vi "Control Panel.vi"(8 "error in (no error)":errorcluster, 11 "Photon Counter SR400 bogus in":refnum<class "Photon Counter SR400.lvclass">) -> (0 "error out":errorcluster, 3 "Photon Counter SR400 bogus out":refnum<class "Photon Counter SR400.lvclass">)   [LabVIEW 2012, in "Photon Counter SR400.lvclass"]
uses:
  Photon Counter SR400.lvclass
  SR400/Public/Typedefs.llb/Gate Mode.ctl
  Photon Counter SR400.lvclass/Photon Counter SR400.ctl
  SR400/SR400.lvlib
  Utility Classes/Readable/Readable.lvclass
panel:
  out "Update visible/hidden":bool
  out "Gate B Mode":T1
  out "Gate A Mode":T1
  in  "stop":bool
  in  "Read to Control":bool
  in  "Read":bool
  in  "Initialize":bool
  out "Gate A % Current":dbl
  out "Gate B % Current":dbl
  in  "Gate B % Set":dbl
  in  "Gate A % Set":dbl
  in  "Gate Width: Time / Percent":bool caption="Gate Width\n        Time / Percent"
  in  "Gate Delay Reference\n        Start / Middle":bool
  in  "Gate B Mode Set":T1
  in  "Gate A Mode Set":T1
  out "Trigger Freq Current":dbl[unit]=42077.399999999994 caption="Trigger Freq"
  in  "Trigger Freq Set":dbl[unit]=42077.399999999994 caption="Trigger Freq."
  in  "Set Time & Freq.":bool
  in  "# Triggers vs Freq/Time":bool
  out "# of Cycles Current":dbl format="%^#_6g"
  in  "# of Cycles Set":dbl format="%^#_6g"
  in  "Set # of Triggers":bool
  in  "Internal / External":bool
  out "cpsB":dbl[unit] caption="CPS B"
  out "cpsA":dbl[unit] caption="CPS A"
  in  "Gate B Width Set":dbl[unit] caption="Gate B Width"
  in  "Gate A Width Set":dbl[unit]
  out "Gate A Width":dbl[unit] format="%^#_6g"
  out "Gate B Width":dbl[unit] format="%^#_6g"
  out "Gate B Delay":dbl[unit]
  out "Gate A Delay":dbl[unit]
  in  "Gate B Delay Set":dbl[unit]
  in  "Gate A Delay Set":dbl[unit]
  in  "Set Gate Delays":bool
  in  "Set Gate Mode":bool
  in  "Set Gate Widths":bool
  in  "Read Channels":bool
  in  "Count Time Set":dbl[unit]
  out "Count Time Current":dbl[unit]=1.0 min=0.0 max=10000.0 step=1.0 format="%#_7g"
  in  "Set Count Time":bool
  out "Photon Counter SR400":refnum<class "Photon Counter SR400.lvclass">
  # "Gates"
  # "Trigger"
  # "Gate A"
  # "Gate B"
  # "Channels"
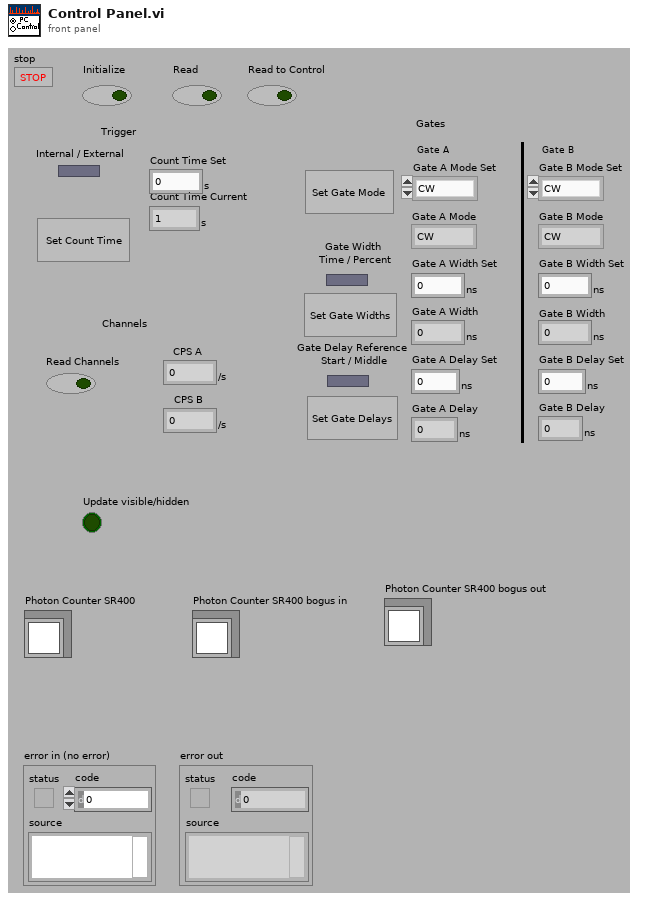
[diagram p1: front panel]
types:
  T1 = typedef "SR400.lvlib/Gate Mode.ctl" = enum16{"CW", "Fixed", "Scan"}
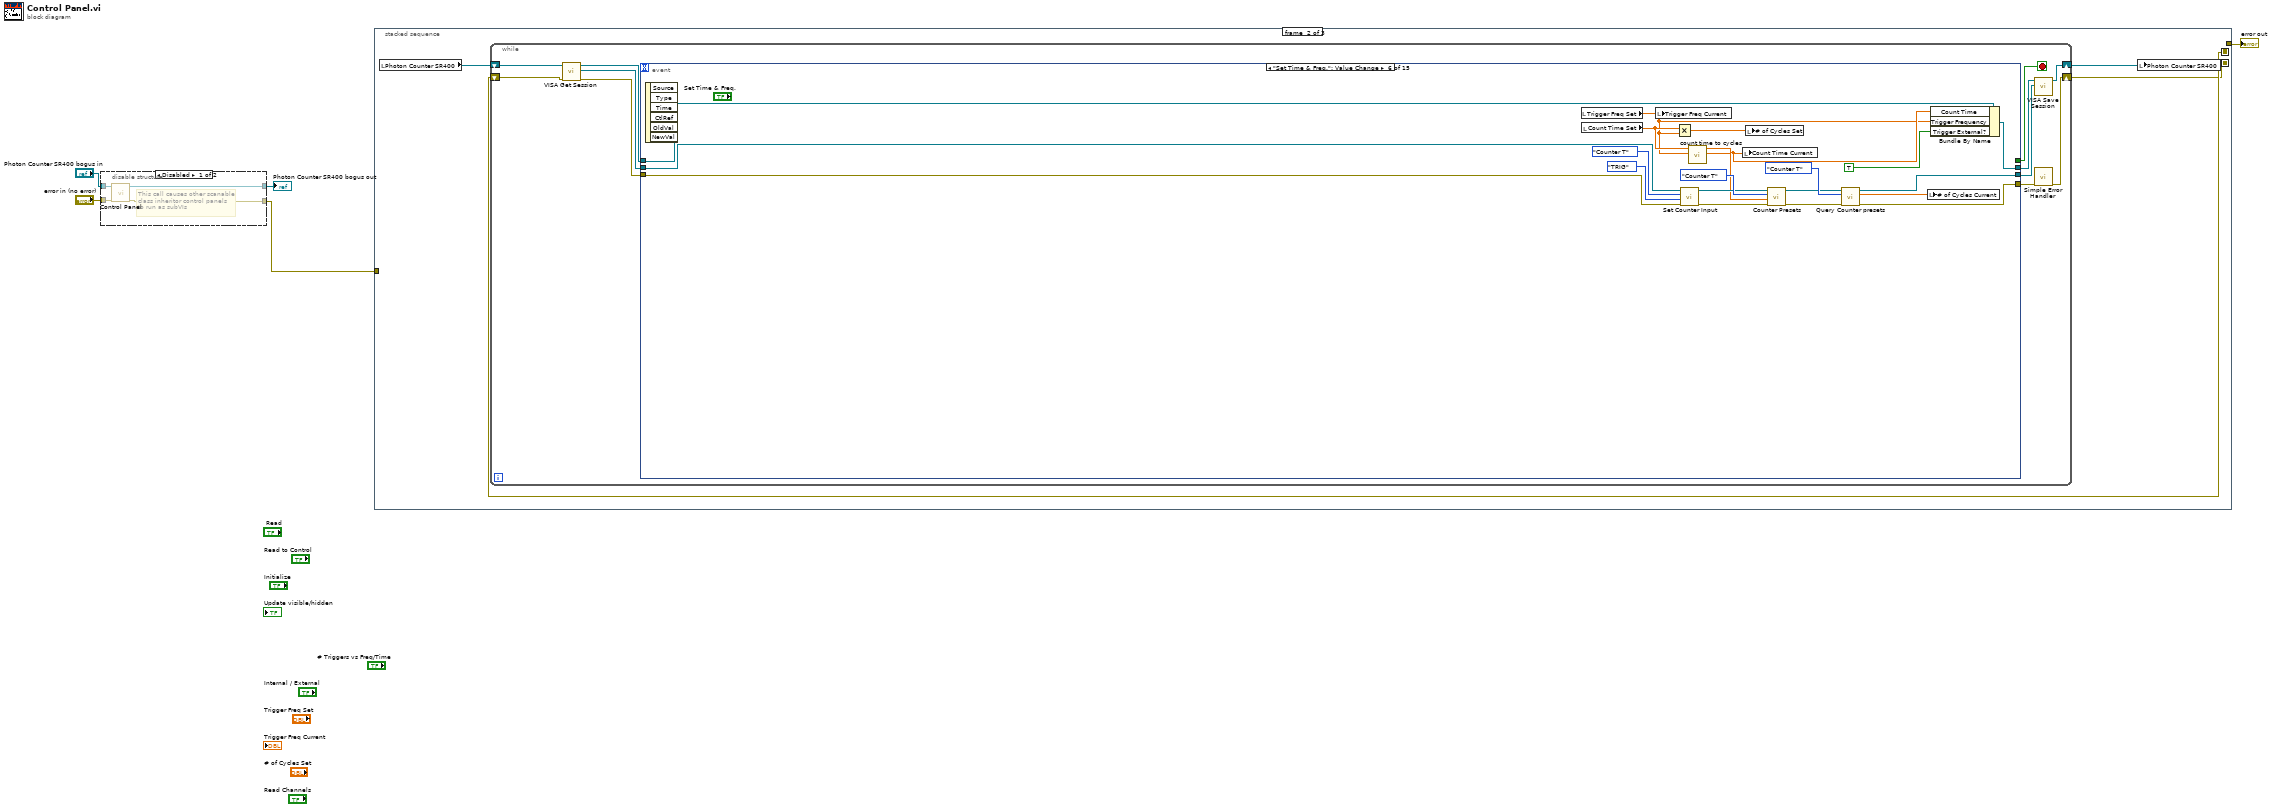
[diagram p0: block diagram]
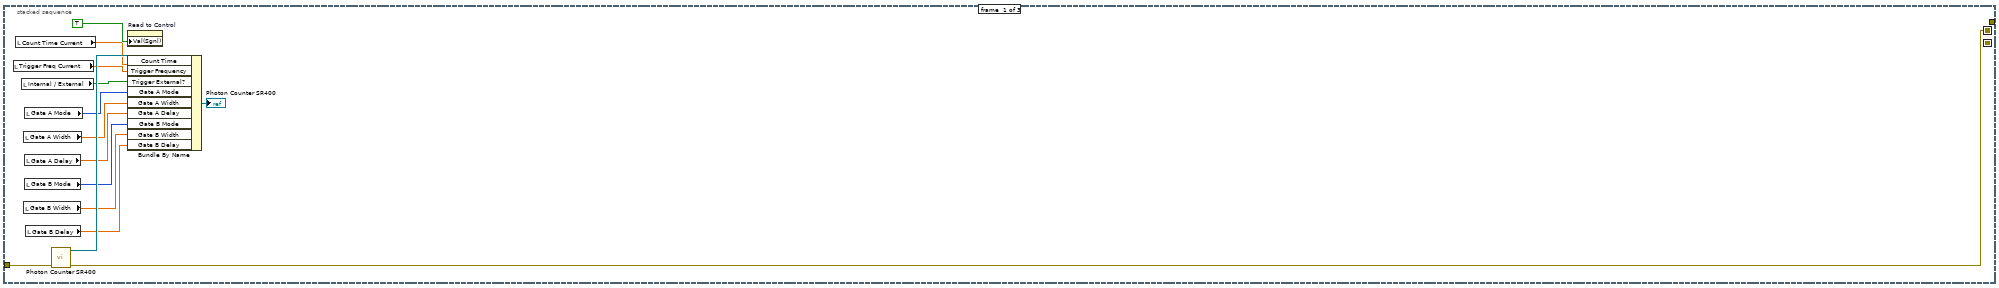
[diagram p3: hidden frame]
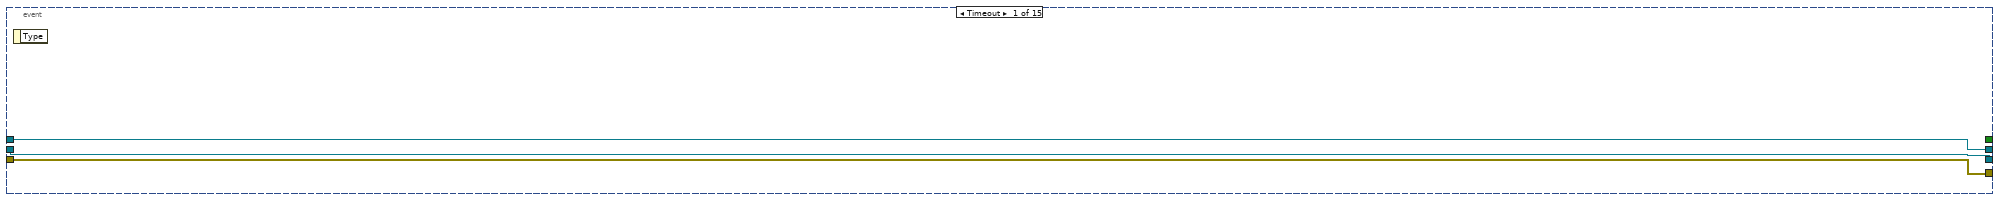
[diagram p4: hidden frame]
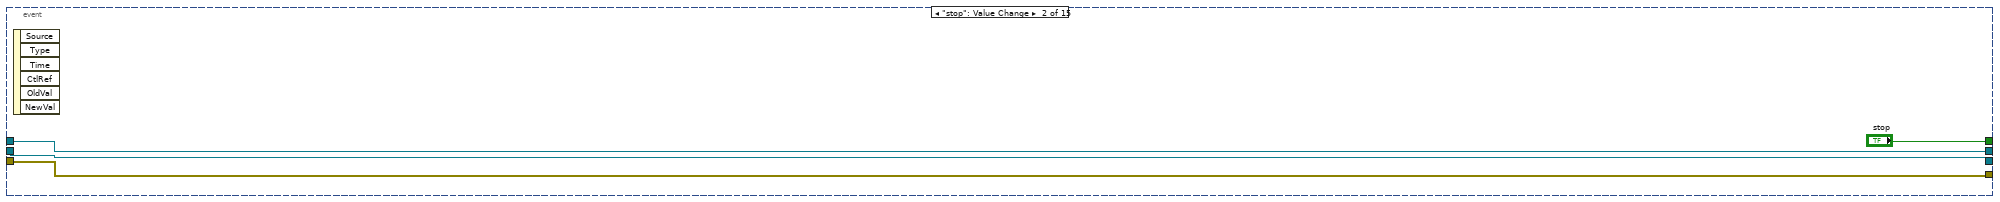
[diagram p5: hidden frame]
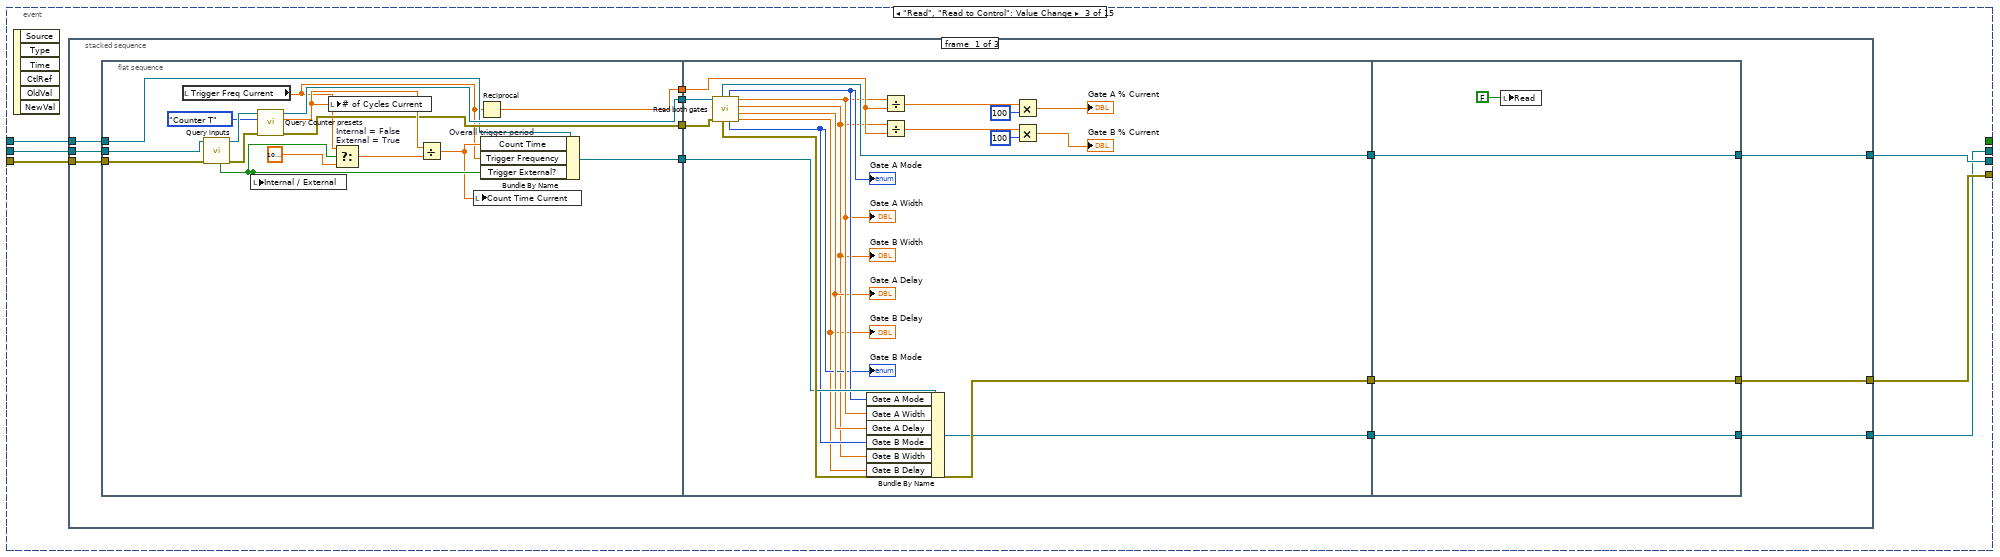
[diagram p6: hidden frame]
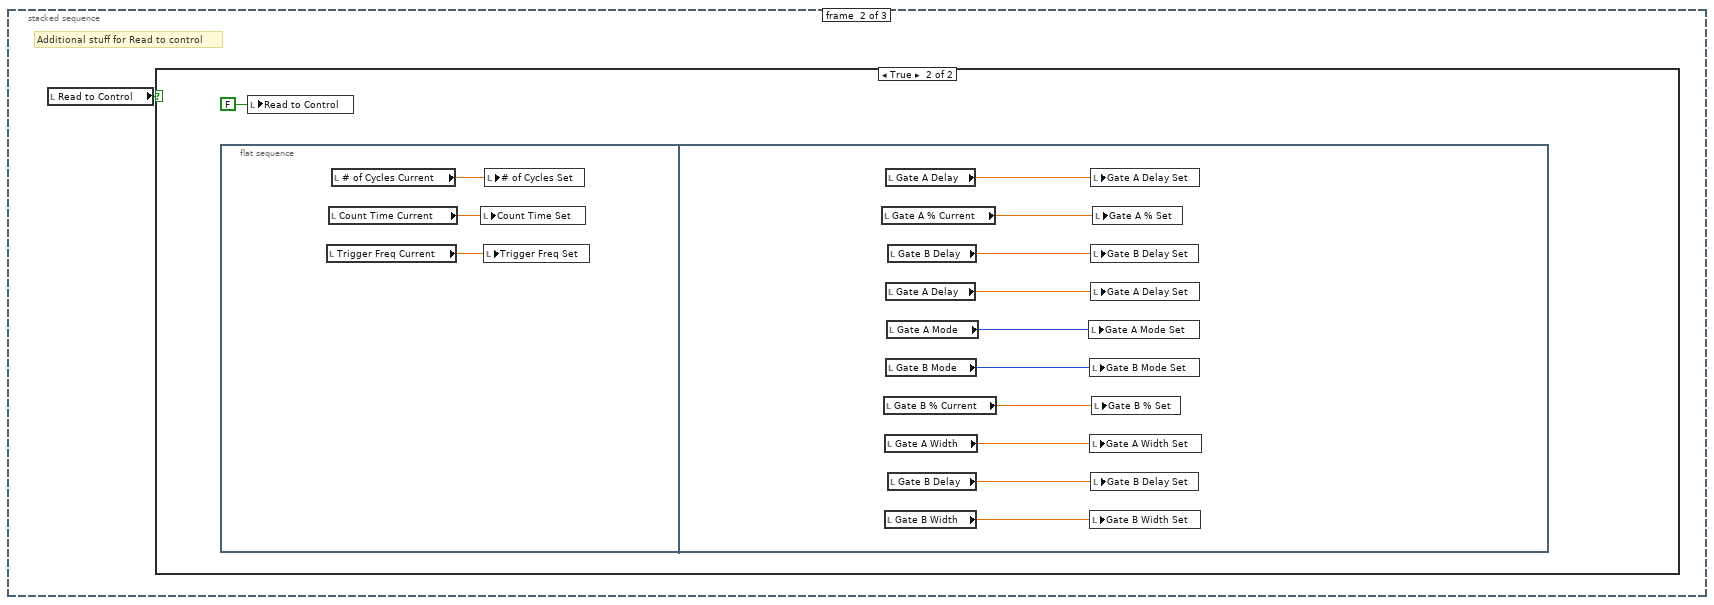
[diagram p7: hidden frame]
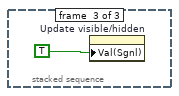
[diagram p9: hidden frame]
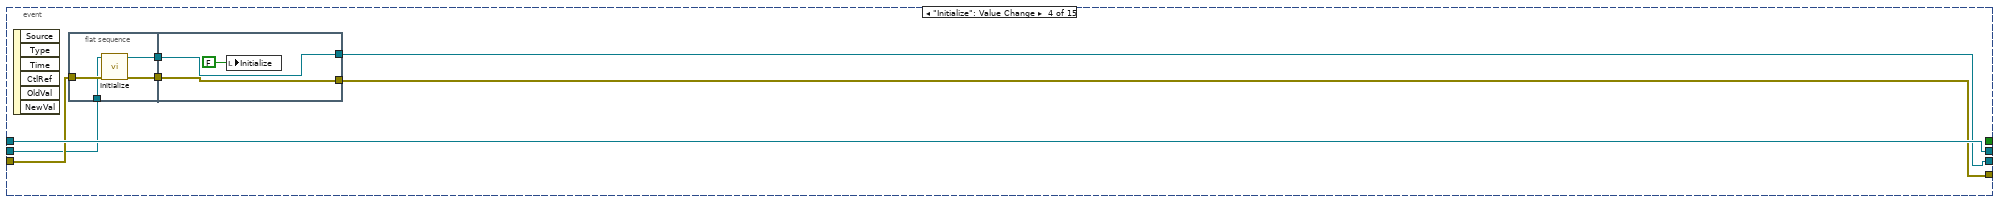
[diagram p10: hidden frame]
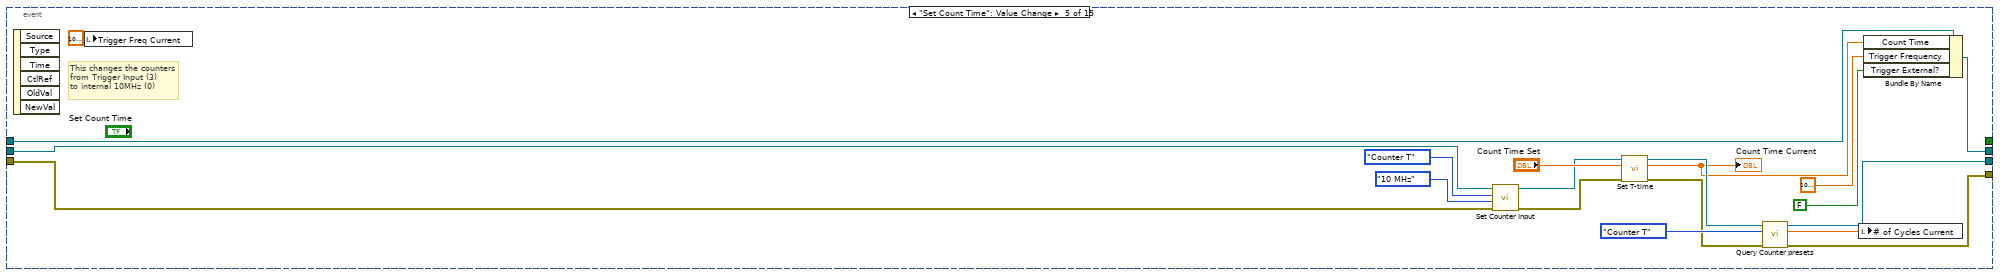
[diagram p11: hidden frame]
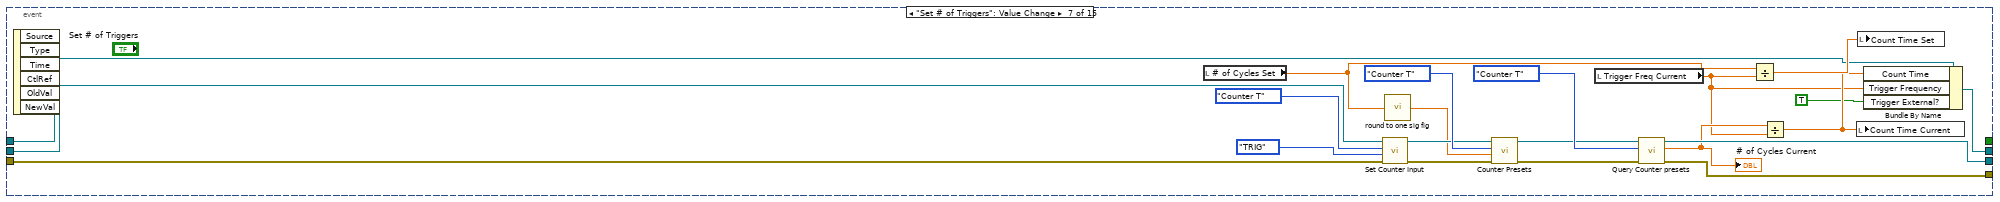
[diagram p12: hidden frame]
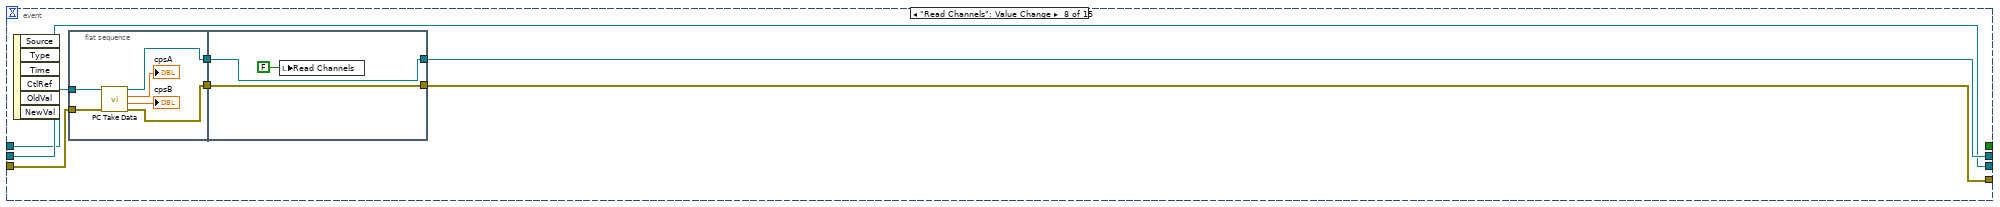
[diagram p13: hidden frame]
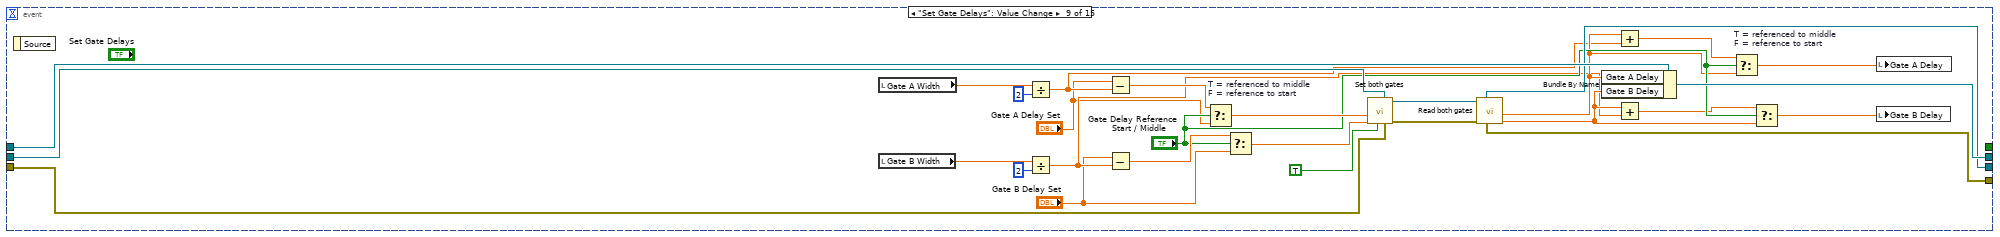
[diagram p14: hidden frame]
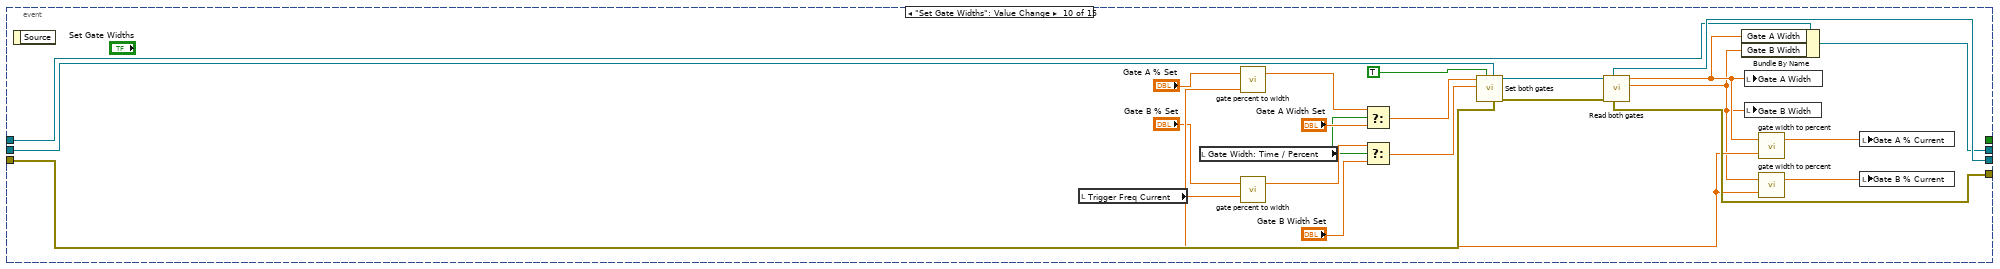
[diagram p15: hidden frame]
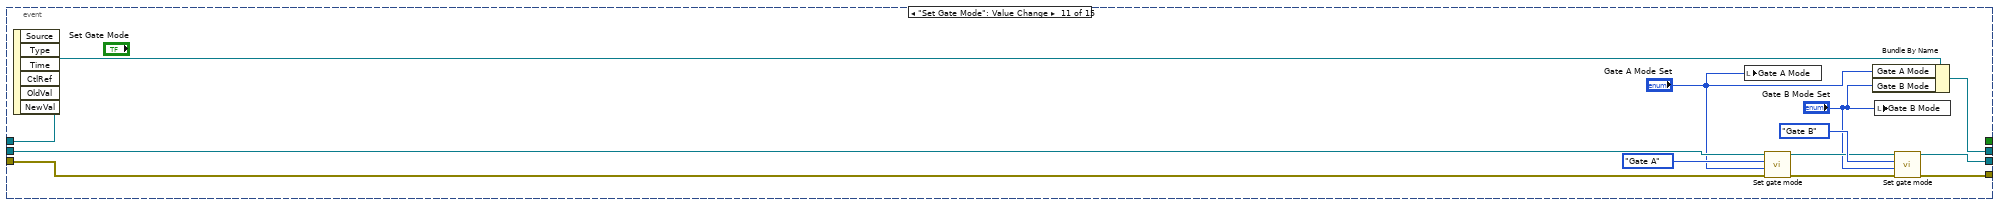
[diagram p16: hidden frame]
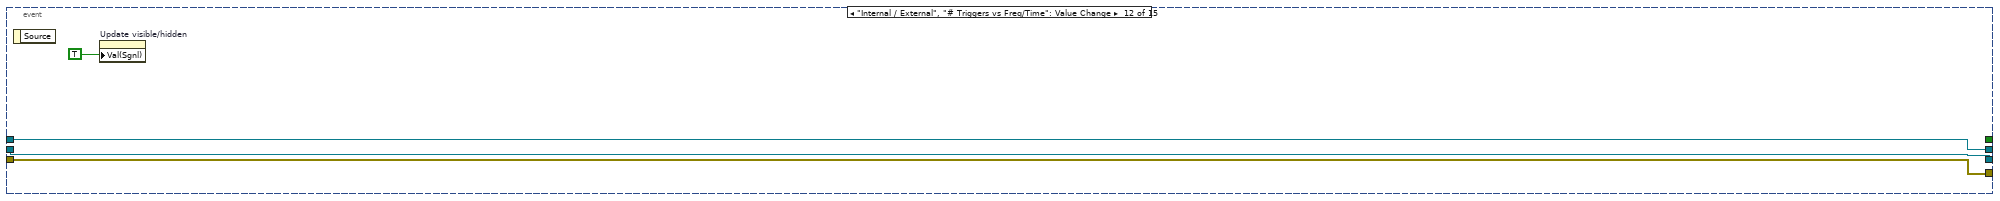
[diagram p17: hidden frame]
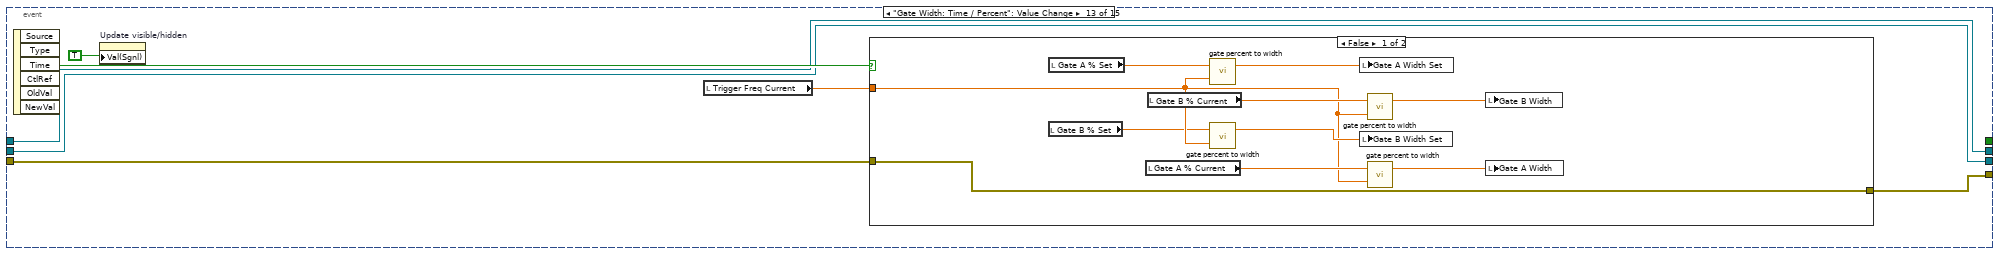
[diagram p18: hidden frame]
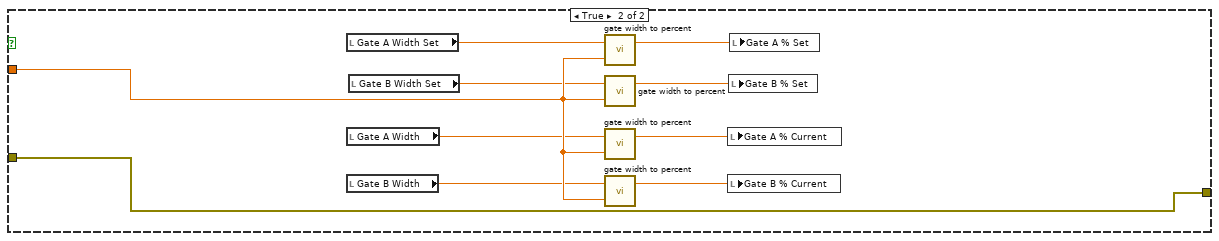
[diagram p19: hidden frame]
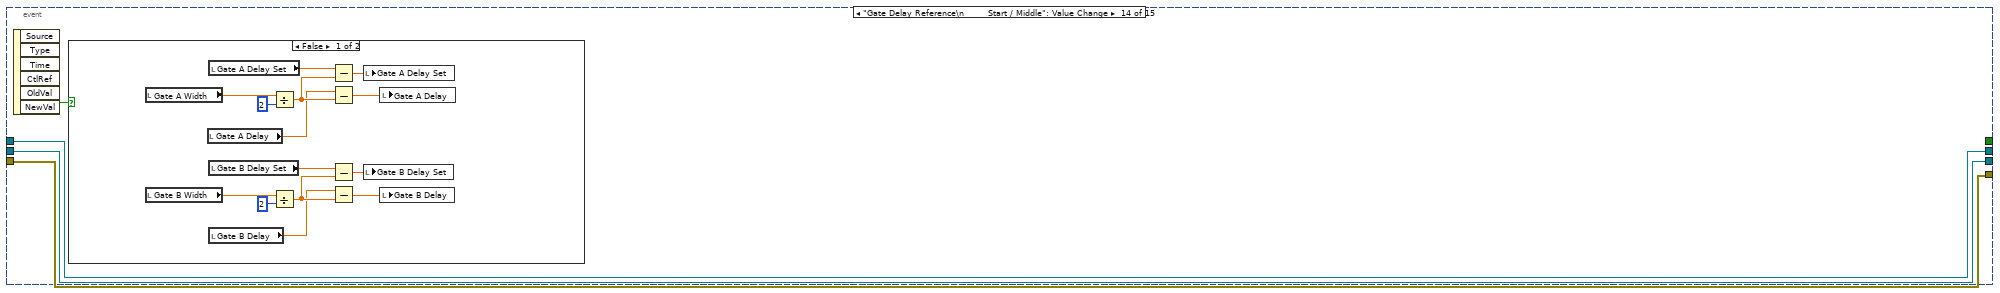
[diagram p20: hidden frame]
diagram:
  n1 = disable-structure shown="Disabled" {
    disable-tunnel: "error in (no error)" -> [w9 w10]
    disable-tunnel: [w8 w10] -> w3
    disable-tunnel: [w7 w11] -> w2
    disable-tunnel: "Photon Counter SR400 bogus in" -> [w6 w11]
    frame Disabled {
      # "This call causes other scanable\nclass inheritor control panels\nto run as subVIs"
      n2 = call-parent "Control Panel.vi"("error in (no error)"=w9, "Instrument in"=w6) -> ("error out"=w8:errorcluster, "Instrument out"=w7:refnum<class "Photon Counter SR400.lvclass">)  [unwired: 8 in]
    }
    frame Enabled {
    }
  }
  "Photon Counter SR400 bogus out" <- w2
  n3 = stacked-sequence {
    seq-local: [w23 _ _] -> [_ w27 _]
    seq-local: [_ w26 _] -> [_ _ w353]
    tunnel: w3 -> [w24 _ _]
    tunnel: [_ _ w352] -> w5
    frame #0 {
      n4 = local read "Trigger Freq Current"() -> (w19:dbl[unit])
      n5 = local read "Count Time Current"() -> (w20:dbl[unit])
      n6 = local read "Internal / External"() -> (w18:bool)
      n7 = local read "Gate A Width"() -> (w16:dbl[unit])
      n8 = local read "Gate B Width"() -> (w13:dbl[unit])
      n9 = local read "Gate A Delay"() -> (w15:dbl[unit])
      n10 = local read "Gate B Mode"() -> (w12:T1)
      n11 = local read "Gate A Mode"() -> (w17:T1)
      n12 = local read "Gate B Delay"() -> (w14:dbl[unit])
      n13 = call "Photon Counter SR400.vi"("error in (no error)"=w24) -> ("error out"=w23:errorcluster, "Photon Counter SR400 out"=w22:refnum<class "Photon Counter SR400.lvclass">)  [unwired: 9 out]
      n14 = Bundle By Name(cluster=w22, "Count Time"=w20, "Trigger Frequency"=w19, "Trigger External?"=w18, "Gate A Mode"=w17, "Gate A Width"=w16, "Gate A Delay"=w15, "Gate B Mode"=w12, "Gate B Width"=w13, "Gate B Delay"=w14) -> (→"Photon Counter SR400":refnum<class "Photon Counter SR400.lvclass">)
      n15 = property on="Read to Control" class="Bool (strict)"("Val(Sgnl)"=TRUE ("Value (Signaling)")) -> ()  [unwired: 2 in, 2 out]
    }
    frame #1 {
      n16 = local read "Photon Counter SR400"() -> (w29:refnum<class "Photon Counter SR400.lvclass">)
      n17 = while {
        shift-right: [w32] -> w28
        shift-left: w29 -> [w37]
        shift-right: [w39] -> w26
        shift-left: w27 -> [w30]
        stop <- w31 stop-if-true
        n18 = call-dynamic "VISA Get Session.vi"("error in (no error)"=w30, "Instrument.lvclass in"=w37) -> ("error out"=w35:errorcluster, "VISA Resource Name"=w38:refnum<visa-resource-name>, "Instrument.lvclass out"=w36:refnum<class "Photon Counter SR400.lvclass">)  [unwired: 7 out]
        n19 = event shown="[5] \"Set Time & Freq.\": Value Change" {
          selector: _ -> [_ _ _ _ _ _ _ _ _ _ _ _ _ _ _]
          dyn-events: _ -> [_ _ _ _ _ _ _ _ _ _ _ _ _ _ _]
          timeout: _ -> [_ _ _ _ _ _ _ _ _ _ _ _ _ _ _]
          tunnel: [w42 w45 w51 w122 w151 w170 w194 w200 w226 w258 w268 w279 w282 w308 w341] -> w34
          tunnel: w35 -> [w41 w44 w53 w127 w142 w164 w186 w203 w240 w259 w272 w278 w280 w307 w340]
          tunnel: [w41 w44 w50 w126 w150 w171 w193 w202 w224 w257 w269 w278 w281 w307 w340] -> w40
          tunnel: w38 -> [w42 w45 w52 w123 w143 w165 w187 w200 w239 w260 w273 w279 w282 w308 w341]
          tunnel: w36 -> [w43 w46 w49 w128 w140 w159 w180 w199 w238 w244 w267 w277 w283 w309 w339]
          tunnel: [w43 w46 w48 w128 w139 w158 w179 w201 w237 w243 w266 w277 w283 w309 w339] -> w33
          tunnel: [_ "stop" _ _ _ _ _ _ _ _ _ _ _ _ _] -> w31
          event Timeout {
            n20 = event-data() -> ()  [unwired: 2 out]
          }
          event "stop": Value Change {
            n21 = event-data() -> ()  [unwired: 7 out]
          }
          event "Read", "Read to Control": Value Change {
            n22 = event-data() -> ()  [unwired: 7 out]
            n23 = stacked-sequence {
              tunnel: w53 -> [w65 _ _]
              tunnel: w52 -> [w66 _ _]
              tunnel: [w61 _ _] -> w51
              tunnel: [w59 _ _] -> w50
              tunnel: w49 -> [w57 _ _]
              tunnel: [w55 _ _] -> w48
              frame #0 {
                n24 = flat-sequence {
                  tunnel: w66 -> [w82]
                  tunnel: w65 -> [w79]
                  tunnel: [w75] -> w64
                  tunnel: [w74] -> w63
                  tunnel: [w73] -> w62
                  tunnel: w57 -> [w71]
                  tunnel: [w67] -> w56
                  tunnel: w64 -> [w95]
                  tunnel: w63 -> [w94]
                  tunnel: w62 -> [w93]
                  tunnel: [w92] -> w60
                  tunnel: [w91] -> w58
                  tunnel: w56 -> [w90]
                  tunnel: [w83] -> w54
                  tunnel: [w104] -> w61
                  tunnel: w60 -> [w104]
                  tunnel: [w103] -> w59
                  tunnel: w58 -> [w103]
                  tunnel: [w102] -> w55
                  tunnel: w54 -> [w102]
                  frame #0 {
                    n25 = local read "Trigger Freq Current"() -> (w68:dbl[unit])
                    n26 = call "Query inputs.vi"("error in (no error)"=w79, "VISA resource name"=w82) -> ("error out"=w80:errorcluster, "VISA resource name out"=w81:refnum<visa-resource-name>, "Externally-triggered?"=w70:bool)  [unwired: 7 out]
                    n27 = local write "Internal / External"(w70) -> ()
                    n28 = call "Query Counter presets.vi"("error in (no error)"=w80, "Counter (Def: T)"=enum16{"Invalid", "Counter B", "Counter T"}."Counter T" ("i (0)"), "VISA resource name"=w81) -> ("error out"=w74:errorcluster, "Number of triggers"=w76:dbl, "VISA resource name out"=w75:refnum<visa-resource-name>)  [unwired: 6 out]
                    n29 = local write "# of Cycles Current"(w76) -> ()
                    n30 = Select "Internal = False\nExternal = True"(t=w68, s=w70, f=dbl[unit] 10000000.0 ("freq")) -> (s? t:f=w77:dbl[unit])
                    n31 = Divide(x=w76, y=w77) -> (x/y=w69:dbl[unit])
                    n32 = local write "Count Time Current"(w69) -> ()
                    n33 = Reciprocal "Overall trigger period"(x=w68) -> (1/x=w73:dbl[unit])
                    n34 = Bundle By Name(cluster=w71, "Count Time"=w69, "Trigger Frequency"=w68, "Trigger External?"=w70) -> (w67:refnum<class "Photon Counter SR400.lvclass">)
                  }
                  frame #1 {
                    n35 = call "Read both gates.vi"("error in (no error)"=w94, "VISA resource name"=w95) -> ("Gate B Delay"=w84:dbl[unit], "Gate A Delay"=w87:dbl[unit], "Gate B Width"=w85:dbl[unit], "Gate A Width"=w88:dbl[unit], "Current mode B"=w86:enum16{"CW", "Fixed", "Scan"}, "Current mode A"=w89:enum16{"CW", "Fixed", "Scan"}, "error out"=w91:errorcluster, "VISA resource name out"=w92:refnum<visa-resource-name>)  [unwired: 2 out]
                    "Gate B Width" <- w85
                    "Gate A Width" <- w88
                    "Gate A Delay" <- w87
                    "Gate B Delay" <- w84
                    "Gate A Mode" <- w89
                    "Gate B Mode" <- w86
                    n36 = Bundle By Name(cluster=w90, "Gate A Mode"=w89, "Gate A Width"=w88, "Gate A Delay"=w87, "Gate B Mode"=w86, "Gate B Width"=w85, "Gate B Delay"=w84) -> (w83:refnum<class "Photon Counter SR400.lvclass">)
                    n37 = Divide(x=w88, y=w93) -> (x/y=w97:dbl)
                    n38 = Divide(x=w85, y=w93) -> (x/y=w99:dbl)
                    n39 = Multiply(x=w97, y=i8 100) -> (x*y=→"Gate A % Current":dbl)
                    n40 = Multiply(x=w99, y=i8 100) -> (x*y=→"Gate B % Current":dbl)
                  }
                  frame #2 {
                    n41 = local write "Read"(FALSE ("Read")) -> ()
                  }
                }
              }
              frame #1 {
                # "Additional stuff for Read to control"
                n42 = local read "Read to Control"() -> (w106:bool)
                n43 = case shown="True" w106 {
                  frame False {
                  }
                  frame True {
                    n44 = flat-sequence {
                      frame #0 {
                        n45 = local read "Trigger Freq Current"() -> (w108:dbl[unit])
                        n46 = local read "Count Time Current"() -> (w110:dbl[unit])
                        n47 = local read "# of Cycles Current"() -> (w109:dbl)
                        n48 = local write "Count Time Set"(w110) -> ()
                        n49 = local write "Trigger Freq Set"(w108) -> ()
                        n50 = local write "# of Cycles Set"(w109) -> ()
                      }
                      frame #1 {
                        n51 = local read "Gate A % Current"() -> (w117:dbl)
                        n52 = local read "Gate B % Current"() -> (w119:dbl)
                        n53 = local read "Gate A Width"() -> (w116:dbl[unit])
                        n54 = local read "Gate B Width"() -> (w111:dbl[unit])
                        n55 = local read "Gate A Delay"() -> (w112:dbl[unit])
                        n56 = local read "Gate A Delay"() -> (w118:dbl[unit])
                        n57 = local read "Gate B Mode"() -> (w115:T1)
                        n58 = local read "Gate A Mode"() -> (w114:T1)
                        n59 = local read "Gate B Delay"() -> (w113:dbl[unit])
                        n60 = local read "Gate B Delay"() -> (w120:dbl[unit])
                        n61 = local write "Gate A Mode Set"(w114) -> ()
                        n62 = local write "Gate B Mode Set"(w115) -> ()
                        n63 = local write "Gate A Width Set"(w116) -> ()
                        n64 = local write "Gate B Width Set"(w111) -> ()
                        n65 = local write "Gate A Delay Set"(w112) -> ()
                        n66 = local write "Gate B Delay Set"(w113) -> ()
                        n67 = local write "Gate A Delay Set"(w118) -> ()
                        n68 = local write "Gate B Delay Set"(w120) -> ()
                        n69 = local write "Gate B % Set"(w119) -> ()
                        n70 = local write "Gate A % Set"(w117) -> ()
                      }
                    }
                    n71 = local write "Read to Control"(FALSE ("Read to Control")) -> ()
                  }
                }
              }
              frame #2 {
                n72 = property on="Update visible/hidden" class="Bool (strict)"("Val(Sgnl)"=TRUE ("Value (Signaling)")) -> ()  [unwired: 2 in, 2 out]
              }
            }
          }
          event "Initialize": Value Change {
            n73 = event-data() -> ()  [unwired: 7 out]
            n74 = flat-sequence {
              tunnel: w127 -> [w132]
              tunnel: [w131] -> w125
              tunnel: [w130] -> w124
              tunnel: w123 -> [w129]
              tunnel: [w134] -> w126
              tunnel: [w135] -> w122
              tunnel: w125 -> [w135]
              tunnel: w124 -> [w134]
              frame #0 {
                n75 = call "Initialize.vi"("errorIN"=w132, "VISA resource name"=w129) -> ("errorOUT"=w130:errorcluster, "VISA resource name out"=w131:refnum<visa-resource-name>)  [unwired: 8 out]
              }
              frame #1 {
                n76 = local write "Initialize"(FALSE ("Re-initialize")) -> ()
              }
            }
          }
          event "Set Count Time": Value Change {
            # "This changes the counters\nfrom Trigger Input (3)\nto internal 10MHz (0)"
            n77 = event-data() -> ()  [unwired: 7 out]
            n78 = local write "Trigger Freq Current"(dbl[unit] 10000000.0 ("freq")) -> ()
            n79 = call "Set Counter Input.vi"("error in (no error)"=w142, "Input (def: 10 MHz)"=enum16{"10 MHz", "INPUT 1", "INPUT 2", "TRIG"}."10 MHz" ("n (0.000000)"), "Counter (def: A)"=enum16{"Counter A", "Counter B", "Counter T"}."Counter T" ("i (0) 2"), "VISA resource name"=w143) -> ("error out"=w145:errorcluster, "VISA resource name out"=w144:refnum<visa-resource-name>)  [unwired: 6 out]
            n80 = call "Set T-time.vi"("errorIN"=w145, "Count Time Set"="Count Time Set", "VISA resource name"=w144) -> ("errorOUT"=w146:errorcluster, "ttimeOUT"=w138:dbl[unit], "VISA resource name out"=w149:refnum<visa-resource-name>)  [unwired: 4 out]
            "Count Time Current" <- w138
            n81 = call "Query Counter presets.vi"("error in (no error)"=w146, "Counter (Def: T)"=enum16{"Invalid", "Counter B", "Counter T"}."Counter T" ("i (0)"), "VISA resource name"=w149) -> ("error out"=w150:errorcluster, "Number of triggers"=w152:dbl, "VISA resource name out"=w151:refnum<visa-resource-name>)  [unwired: 6 out]
            n82 = local write "# of Cycles Current"(w152) -> ()
            n83 = Bundle By Name(cluster=w140, "Count Time"=w138, "Trigger Frequency"=dbl[unit] 10000000.0, "Trigger External?"=FALSE) -> (w139:refnum<class "Photon Counter SR400.lvclass">)
          }
          event "Set Time & Freq.": Value Change {
            n84 = event-data() -> ()  [unwired: 7 out]
            n85 = local read "Trigger Freq Set"() -> (w155:dbl[unit])
            n86 = local read "Count Time Set"() -> (w160:dbl[unit])
            n87 = local write "Trigger Freq Current"(w155) -> ()
            n88 = Multiply(x=w160, y=w155) -> (x*y=w161:dbl)
            n89 = call "Set Counter Input.vi"("error in (no error)"=w164, "Input (def: 10 MHz)"=enum16{"10 MHz", "INPUT 1", "INPUT 2", "TRIG"}."TRIG" ("n (0.000000)"), "Counter (def: A)"=enum16{"Counter A", "Counter B", "Counter T"}."Counter T" ("i (0) 2"), "VISA resource name"=w165) -> ("error out"=w166:errorcluster, "VISA resource name out"=w167:refnum<visa-resource-name>)  [unwired: 6 out]
            n90 = call "count time to cycles.vi"("Trigger Freq"=w155, "Count Time Set"=w160) -> ("Count Time Current"=w156:dbl[unit], "Number of triggers"=w162:dbl)  [unwired: 1 in, 3 out]
            n91 = local write "Count Time Current"(w156) -> ()
            n92 = local write "# of Cycles Set"(w161) -> ()
            n93 = call "Counter Presets.vi"("error in (no error)"=w166, "Number of triggers"=w162, "Counter (Def: T)"=enum16{"Invalid", "Counter B", "Counter T"}."Counter T" ("i (0) 2"), "VISA resource name"=w167) -> ("error out"=w172:errorcluster, "VISA resource name out"=w169:refnum<visa-resource-name>)  [unwired: 6 out]
            n94 = call "Query Counter presets.vi"("error in (no error)"=w172, "Counter (Def: T)"=enum16{"Invalid", "Counter B", "Counter T"}."Counter T" ("i (0)"), "VISA resource name"=w169) -> ("error out"=w171:errorcluster, "Number of triggers"=w173:dbl, "VISA resource name out"=w170:refnum<visa-resource-name>)  [unwired: 6 out]
            n95 = local write "# of Cycles Current"(w173) -> ()
            n96 = Bundle By Name(cluster=w159, "Count Time"=w156, "Trigger Frequency"=w155, "Trigger External?"=TRUE) -> (w158:refnum<class "Photon Counter SR400.lvclass">)
          }
          event "Set # of Triggers": Value Change {
            n97 = event-data() -> ()  [unwired: 7 out]
            n98 = local read "# of Cycles Set"() -> (w184:dbl)
            n99 = call "Set Counter Input.vi"("error in (no error)"=w186, "Input (def: 10 MHz)"=enum16{"10 MHz", "INPUT 1", "INPUT 2", "TRIG"}."TRIG" ("n (0.000000)"), "Counter (def: A)"=enum16{"Counter A", "Counter B", "Counter T"}."Counter T" ("i (0) 2"), "VISA resource name"=w187) -> ("error out"=w188:errorcluster, "VISA resource name out"=w189:refnum<visa-resource-name>)  [unwired: 6 out]
            n100 = call "round to one sig fig.vi"("input number"=w184) -> ("rounded to 1 sig fig"=w182:dbl)
            n101 = call "Counter Presets.vi"("error in (no error)"=w188, "Number of triggers"=w182, "Counter (Def: T)"=enum16{"Invalid", "Counter B", "Counter T"}."Counter T" ("i (0) 2"), "VISA resource name"=w189) -> ("error out"=w192:errorcluster, "VISA resource name out"=w191:refnum<visa-resource-name>)  [unwired: 6 out]
            n102 = local read "Trigger Freq Current"() -> (w176:dbl[unit])
            n103 = call "Query Counter presets.vi"("error in (no error)"=w192, "Counter (Def: T)"=enum16{"Invalid", "Counter B", "Counter T"}."Counter T" ("i (0)"), "VISA resource name"=w191) -> ("error out"=w193:errorcluster, "Number of triggers"=w181:dbl, "VISA resource name out"=w194:refnum<visa-resource-name>)  [unwired: 6 out]
            "# of Cycles Current" <- w181
            n104 = Divide(x=w184, y=w176) -> (x/y=w183:dbl[unit])
            n105 = Divide(x=w181, y=w176) -> (x/y=w178:dbl[unit])
            n106 = local write "Count Time Current"(w178) -> ()
            n107 = local write "Count Time Set"(w183) -> ()
            n108 = Bundle By Name(cluster=w180, "Count Time"=w178, "Trigger Frequency"=w176, "Trigger External?"=TRUE) -> (w179:refnum<class "Photon Counter SR400.lvclass">)
          }
          event "Read Channels": Value Change {
            n109 = event-data() -> ()  [unwired: 7 out]
            n110 = flat-sequence {
              tunnel: w203 -> [w209]
              tunnel: w199 -> [w204]
              tunnel: [w208] -> w198
              tunnel: [w205] -> w197
              tunnel: [w211] -> w201
              tunnel: [w212] -> w202
              tunnel: w198 -> [w212]
              tunnel: w197 -> [w211]
              frame #0 {
                n111 = call "PC Take Data.vi"("error in (no error)"=w209, "Photon Counter SR400 in"=w204) -> ("error out"=w208:errorcluster, "CPS B"=→"cpsB":dbl[unit], "CPS A"=→"cpsA":dbl[unit], "Photon Counter SR400 out"=w205:refnum<class "Photon Counter SR400.lvclass">)  [unwired: 2 in, 4 out]
              }
              frame #1 {
                n112 = local write "Read Channels"(FALSE ("Read Channels")) -> ()
              }
            }
          }
          event "Set Gate Delays": Value Change {
            n113 = event-data() -> ()  [unwired: 2 out]
            n114 = local read "Gate A Width"() -> (w235:dbl[unit])
            n115 = local read "Gate B Width"() -> (w234:dbl[unit])
            n116 = Divide(x=w235, y=2) -> (x/y=w214:dbl[unit])
            n117 = Divide(x=w234, y=2) -> (x/y=w216:dbl[unit])
            n118 = Subtract(x="Gate A Delay Set", y=w214) -> (x-y=w231:dbl[unit])
            n119 = Subtract(x="Gate B Delay Set", y=w216) -> (x-y=w229:dbl[unit])
            n120 = Select "T = referenced to middle\nF = reference to start"(t=w231, s="Gate Delay Reference\n        Start / Middle", f="Gate A Delay Set") -> (s? t:f=w228:dbl[unit])
            n121 = Select(t=w229, s="Gate Delay Reference\n        Start / Middle", f="Gate B Delay Set") -> (s? t:f=w230:dbl[unit])
            n122 = call "Set both gates.vi"("Error In"=w240, "VISA resource name"=w239, "Set Delay?"=TRUE, "gatedelayoffsetB"=w230, "gatedelayoffsetA"=w228) -> ("Error Out"=w225:errorcluster, "VISA resource name out"=w227:refnum<visa-resource-name>)  [unwired: 3 in, 2 out]
            n123 = call "Read both gates.vi"("error in (no error)"=w225, "VISA resource name"=w227) -> ("Gate B Delay"=w221:dbl[unit], "Gate A Delay"=w222:dbl[unit], "error out"=w224:errorcluster, "VISA resource name out"=w226:refnum<visa-resource-name>)  [unwired: 6 out]
            n124 = Bundle By Name(cluster=w238, "Gate A Delay"=w222, "Gate B Delay"=w221) -> (w237:refnum<class "Photon Counter SR400.lvclass">)
            n125 = Add(x=w222, y=w214) -> (x+y=w220:dbl[unit])
            n126 = Add(x=w221, y=w216) -> (x+y=w219:dbl[unit])
            n127 = Select "T = referenced to middle\nF = reference to start"(t=w220, s="Gate Delay Reference\n        Start / Middle", f=w222) -> (s? t:f=w218:dbl[unit])
            n128 = Select(t=w219, s="Gate Delay Reference\n        Start / Middle", f=w221) -> (s? t:f=w217:dbl[unit])
            n129 = local write "Gate A Delay"(w218) -> ()
            n130 = local write "Gate B Delay"(w217) -> ()
          }
          event "Set Gate Widths": Value Change {
            n131 = event-data() -> ()  [unwired: 2 out]
            n132 = local read "Trigger Freq Current"() -> (w254:dbl[unit])
            n133 = local read "Gate Width: Time / Percent"() -> (w247:bool)
            n134 = call "gate percent to width.vi"("Trigger Freq"=w254, "Gate %"="Gate A % Set") -> ("Gate width"=w249:dbl[unit])  [unwired: 1 out]
            n135 = call "gate percent to width.vi"("Trigger Freq"=w254, "Gate %"="Gate B % Set") -> ("Gate width"=w248:dbl[unit])  [unwired: 1 out]
            n136 = Select(t=w249, s=w247, f="Gate A Width Set") -> (s? t:f=w250:dbl[unit])
            n137 = Select(t=w248, s=w247, f="Gate B Width Set") -> (s? t:f=w245:dbl[unit])
            n138 = call "Set both gates.vi"("Error In"=w259, "VISA resource name"=w260, "Set Width?"=TRUE, "Gate B Width"=w245, "Gate A Width"=w250) -> ("Error Out"=w263:errorcluster, "VISA resource name out"=w262:refnum<visa-resource-name>)  [unwired: 3 in, 2 out]
            n139 = call "Read both gates.vi"("error in (no error)"=w263, "VISA resource name"=w262) -> ("Gate B Width"=w241:dbl[unit], "Gate A Width"=w242:dbl[unit], "error out"=w257:errorcluster, "VISA resource name out"=w258:refnum<visa-resource-name>)  [unwired: 6 out]
            n140 = Bundle By Name(cluster=w244, "Gate A Width"=w242, "Gate B Width"=w241) -> (w243:refnum<class "Photon Counter SR400.lvclass">)
            n141 = local write "Gate A Width"(w242) -> ()
            n142 = local write "Gate B Width"(w241) -> ()
            n143 = call "gate width to percent.vi"("Trigger Freq"=w254, "Gate width"=w242) -> ("Gate %"=w255:dbl)  [unwired: 1 out]
            n144 = call "gate width to percent.vi"("Trigger Freq"=w254, "Gate width"=w241) -> ("Gate %"=w256:dbl)  [unwired: 1 out]
            n145 = local write "Gate A % Current"(w255) -> ()
            n146 = local write "Gate B % Current"(w256) -> ()
          }
          event "Set Gate Mode": Value Change {
            n147 = event-data() -> ()  [unwired: 7 out]
            n148 = local write "Gate A Mode"("Gate A Mode Set") -> ()
            n149 = call "Set gate mode.vi"("error in (no error)"=w272, "Mode (def: CW)"="Gate A Mode Set", "Gate (def: A)"=enum16{"Gate A", "Gate B"}."Gate A" ("i (0)"), "VISA resource name"=w273) -> ("error out"=w271:errorcluster, "VISA resource name out"=w270:refnum<visa-resource-name>)  [unwired: 6 out]
            n150 = Bundle By Name(cluster=w267, "Gate A Mode"="Gate A Mode Set", "Gate B Mode"="Gate B Mode Set") -> (w266:refnum<class "Photon Counter SR400.lvclass">)
            n151 = local write "Gate B Mode"("Gate B Mode Set") -> ()
            n152 = call "Set gate mode.vi"("error in (no error)"=w271, "Mode (def: CW)"="Gate B Mode Set", "Gate (def: A)"=enum16{"Gate A", "Gate B"}."Gate B" ("i (0)"), "VISA resource name"=w270) -> ("error out"=w269:errorcluster, "VISA resource name out"=w268:refnum<visa-resource-name>)  [unwired: 6 out]
          }
          event "Internal / External", "# Triggers vs Freq/Time": Value Change {
            n153 = event-data() -> ()  [unwired: 2 out]
            n154 = property on="Update visible/hidden" class="Bool (strict)"("Val(Sgnl)"=TRUE ("Value (Signaling)")) -> ()  [unwired: 2 in, 2 out]
          }
          event "Gate Width: Time / Percent": Value Change {
            n155 = event-data() -> ("NewVal"=w284:bool)  [unwired: 6 out]
            n156 = property on="Update visible/hidden" class="Bool (strict)"("Val(Sgnl)"=TRUE ("Value (Signaling)")) -> ()  [unwired: 2 in, 2 out]
            n157 = local read "Trigger Freq Current"() -> (w285:dbl[unit])
            n158 = case shown="False" w284 {
              tunnel: w285 -> [w290 w306]
              tunnel: [w287 w297] -> w281
              tunnel: w280 -> [w287 w297]
              frame False {
                n159 = local read "Gate B % Set"() -> (w289:dbl)
                n160 = local read "Gate A % Set"() -> (w288:dbl)
                n161 = local read "Gate A % Current"() -> (w294:dbl)
                n162 = local read "Gate B % Current"() -> (w293:dbl)
                n163 = call "gate percent to width.vi"("Trigger Freq"=w290, "Gate %"=w288) -> ("Gate width"=w296:dbl[unit])  [unwired: 1 out]
                n164 = call "gate percent to width.vi"("Trigger Freq"=w290, "Gate %"=w289) -> ("Gate width"=w295:dbl[unit])  [unwired: 1 out]
                n165 = local write "Gate A Width Set"(w296) -> ()
                n166 = local write "Gate B Width Set"(w295) -> ()
                n167 = call "gate percent to width.vi"("Trigger Freq"=w290, "Gate %"=w293) -> ("Gate width"=w291:dbl[unit])  [unwired: 1 out]
                n168 = call "gate percent to width.vi"("Trigger Freq"=w290, "Gate %"=w294) -> ("Gate width"=w292:dbl[unit])  [unwired: 1 out]
                n169 = local write "Gate B Width"(w291) -> ()
                n170 = local write "Gate A Width"(w292) -> ()
              }
              frame True {
                n171 = local read "Gate A Width Set"() -> (w305:dbl[unit])
                n172 = local read "Gate A Width"() -> (w301:dbl[unit])
                n173 = local read "Gate B Width"() -> (w299:dbl[unit])
                n174 = local read "Gate B Width Set"() -> (w303:dbl[unit])
                n175 = call "gate width to percent.vi"("Trigger Freq"=w306, "Gate width"=w305) -> ("Gate %"=w304:dbl)  [unwired: 1 out]
                n176 = call "gate width to percent.vi"("Trigger Freq"=w306, "Gate width"=w303) -> ("Gate %"=w302:dbl)  [unwired: 1 out]
                n177 = call "gate width to percent.vi"("Trigger Freq"=w306, "Gate width"=w301) -> ("Gate %"=w300:dbl)  [unwired: 1 out]
                n178 = call "gate width to percent.vi"("Trigger Freq"=w306, "Gate width"=w299) -> ("Gate %"=w298:dbl)  [unwired: 1 out]
                n179 = local write "Gate A % Current"(w300) -> ()
                n180 = local write "Gate B % Current"(w298) -> ()
                n181 = local write "Gate B % Set"(w302) -> ()
                n182 = local write "Gate A % Set"(w304) -> ()
              }
            }
          }
          event "Gate Delay Reference\n        Start / Middle": Value Change {
            n183 = event-data() -> ("NewVal"=w310:bool)  [unwired: 6 out]
            n184 = case shown="False" w310 {
              frame False {
                n185 = local read "Gate A Width"() -> (w324:dbl[unit])
                n186 = local read "Gate B Width"() -> (w321:dbl[unit])
                n187 = local read "Gate A Delay"() -> (w317:dbl[unit])
                n188 = local read "Gate A Delay Set"() -> (w319:dbl[unit])
                n189 = local read "Gate B Delay Set"() -> (w314:dbl[unit])
                n190 = local read "Gate B Delay"() -> (w312:dbl[unit])
                n191 = Divide(x=w324, y=2) -> (x/y=w320:dbl[unit])
                n192 = Divide(x=w321, y=2) -> (x/y=w315:dbl[unit])
                n193 = Subtract(x=w319, y=w320) -> (x-y=w318:dbl[unit])
                n194 = Subtract(x=w317, y=w320) -> (x-y=w316:dbl[unit])
                n195 = Subtract(x=w314, y=w315) -> (x-y=w313:dbl[unit])
                n196 = Subtract(x=w312, y=w315) -> (x-y=w311:dbl[unit])
                n197 = local write "Gate A Delay Set"(w318) -> ()
                n198 = local write "Gate B Delay Set"(w313) -> ()
                n199 = local write "Gate A Delay"(w316) -> ()
                n200 = local write "Gate B Delay"(w311) -> ()
              }
              frame True {
                n201 = local read "Gate A Width"() -> (w338:dbl[unit])
                n202 = local read "Gate B Width"() -> (w335:dbl[unit])
                n203 = local read "Gate A Delay"() -> (w331:dbl[unit])
                n204 = local read "Gate A Delay Set"() -> (w333:dbl[unit])
                n205 = local read "Gate B Delay Set"() -> (w328:dbl[unit])
                n206 = local read "Gate B Delay"() -> (w326:dbl[unit])
                n207 = Divide(x=w338, y=2) -> (x/y=w334:dbl[unit])
                n208 = Divide(x=w335, y=2) -> (x/y=w329:dbl[unit])
                n209 = Add(x=w333, y=w334) -> (x+y=w332:dbl[unit])
                n210 = Add(x=w331, y=w334) -> (x+y=w330:dbl[unit])
                n211 = Add(x=w328, y=w329) -> (x+y=w327:dbl[unit])
                n212 = Add(x=w326, y=w329) -> (x+y=w325:dbl[unit])
                n213 = local write "Gate A Delay Set"(w332) -> ()
                n214 = local write "Gate B Delay Set"(w327) -> ()
                n215 = local write "Gate A Delay"(w330) -> ()
                n216 = local write "Gate B Delay"(w325) -> ()
              }
            }
          }
          event "Update visible/hidden": Value Change {
            n217 = event-data() -> ()  [unwired: 7 out]
            n218 = flat-sequence {
              frame #0 {
                n219 = property on="Gate A % Set" class="DigNum (strict)"("Visible"="Gate Width: Time / Percent") -> ()  [unwired: 2 in, 2 out]
                n220 = property on="Gate B % Set" class="DigNum (strict)"("Visible"="Gate Width: Time / Percent") -> ()  [unwired: 2 in, 2 out]
                n221 = property on="Gate A % Current" class="DigNum (strict)"("Visible"="Gate Width: Time / Percent") -> ()  [unwired: 2 in, 2 out]
                n222 = property on="Gate B % Current" class="DigNum (strict)"("Visible"="Gate Width: Time / Percent") -> ()  [unwired: 2 in, 2 out]
                n223 = Not(x="Gate Width: Time / Percent") -> (.not. x?=w344:bool)
                n224 = property on="Gate B Width Set" class="DigNum (strict)"("Visible"=w344) -> ()  [unwired: 2 in, 2 out]
                n225 = property on="Gate B Width" class="DigNum (strict)"("Visible"=w344) -> ()  [unwired: 2 in, 2 out]
                n226 = property on="Gate A Width" class="DigNum (strict)"("Visible"=w344) -> ()  [unwired: 2 in, 2 out]
                n227 = property on="Gate A Width Set" class="DigNum (strict)"("Visible"=w344) -> ()  [unwired: 2 in, 2 out]
              }
              frame #1 {
                n228 = local read "# Triggers vs Freq/Time"() -> (w346:bool)
                n229 = local read "Internal / External"() -> (w347:bool)
                n230 = property on="# Triggers vs Freq/Time" class="Bool (strict)"("Visible"=w347) -> ()  [unwired: 2 in, 2 out]
                n231 = Not(x=w346) -> (.not. x?=w348:bool)
                n232 = Not(x=w347) -> (.not. x?=w345:bool)
                n233 = And(x=w347, y=w346) -> (x .and. y?=w350:bool)
                n234 = Or(x=w345, y=w346) -> (x .or. y?=w351:bool)
                n235 = property on="Set Count Time" class="Bool"("Visible"=w345) -> ()  [unwired: 2 in, 2 out]
                n236 = property on="Trigger Freq Set" class="DigNum (strict)"("Visible"=w350) -> ()  [unwired: 2 in, 2 out]
                n237 = property on="Set Time & Freq." class="Bool"("Visible"=w350) -> ()  [unwired: 2 in, 2 out]
                n238 = property on="Trigger Freq Current" class="DigNum (strict)"("Visible"=w350) -> ()  [unwired: 2 in, 2 out]
                n239 = And(x=w347, y=w348) -> (x .and. y?=w349:bool)
                n240 = property on="Count Time Current" class="DigNum (strict)"("Visible"=w351) -> ()  [unwired: 2 in, 2 out]
                n241 = property on="Count Time Set" class="DigNum (strict)"("Visible"=w351) -> ()  [unwired: 2 in, 2 out]
                n242 = property on="# of Cycles Set" class="DigNum (strict)"("Visible"=w349) -> ()  [unwired: 2 in, 2 out]
                n243 = property on="# of Cycles Current" class="DigNum (strict)"("Visible"=w349) -> ()  [unwired: 2 in, 2 out]
                n244 = property on="Set # of Triggers" class="Bool"("Visible"=w349) -> ()  [unwired: 2 in, 2 out]
              }
            }
            n245 = local write "Update visible/hidden"(FALSE ("Update visiible/hidden")) -> ()
          }
        }
        n246 = call-dynamic "VISA Save Session.vi"("VISA Resource Name"=w34, "Instrument.lvclass in"=w33) -> ("Instrument.lvclass out"=w32:refnum<class "Photon Counter SR400.lvclass">)  [unwired: 1 in, 8 out]
        n247 = call <vilib>:"Simple Error Handler.vi"("error in (no error)"=w40) -> ("error out"=w39:errorcluster)  [unwired: 1 in, 7 out]
      }
      n248 = local write "Photon Counter SR400"(w28) -> ()
    }
    frame #2 {
      n249 = local read "Photon Counter SR400"() -> (w354:refnum<class "Photon Counter SR400.lvclass">)
      n250 = call-dynamic "_Destroy.vi"("error in (no error)"=w353, "Photon Counter SR400 in"=w354) -> ("error out"=w352:errorcluster)  [unwired: 9 out]
    }
  }
  "error out" <- w5
